vi "Construct Data Replay Control String.vi"(10 "Control String Info":T1, 11 "Control Name":string) -> (3 "Control":string)   [LabVIEW 2011, in "Engine Sim System Explorer.lvlib"]
uses:
  Engine Sim System Explorer.lvlib
  TypeDefs/DataReplayCtrlStringInfo.ctl
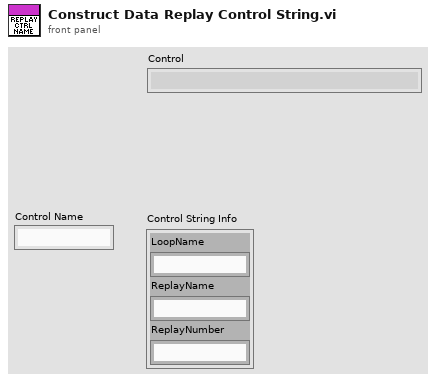
[diagram p1: front panel]
types:
  T1 = typedef "Engine Sim System Explorer.lvlib/DataReplayCtrlStringInfo.ctl" = cluster{"LoopName":string, "ReplayName":string, "ReplayNumber":string}
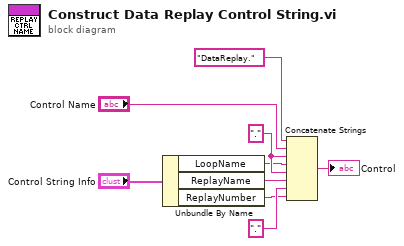
[diagram p0: block diagram]
diagram:
  w5 = "." ("string")
  n1 = Unbundle By Name("Control String Info") -> ("LoopName"=w3:string, "ReplayName"=w2:string, "ReplayNumber"=w1:string)
  n2 = Concatenate Strings("DataReplay." ("string"), "Control Name", w5, w3, w5, w2, ".", w1) -> (→"Control":string)
